vi "Change Password.vi"(8 "error in":errorcluster, 10 "New Password":string, 11 "User Name":string) -> (0 "error out":errorcluster)   [LabVIEW 2022 SP3]
uses:
  <vilib>/Utility/file.llb/Read Delimited Spreadsheet (string).vi
  <vilib>/Utility/file.llb/Write Delimited Spreadsheet (string).vi
panel:
  out "output array 2":string[](array[string])
  out "index of element":i32
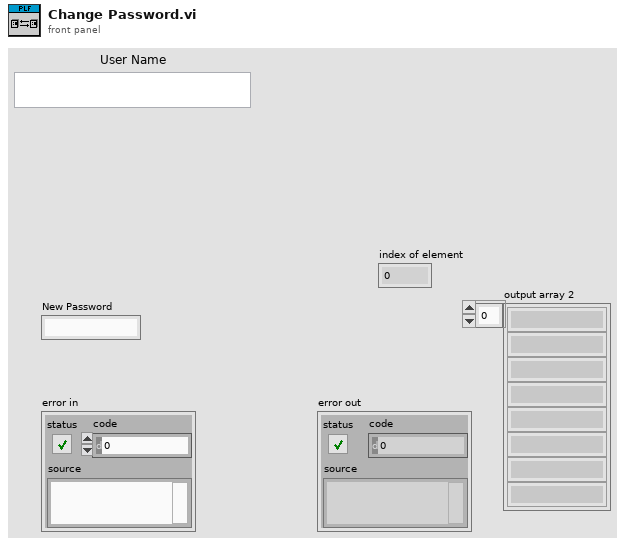
[diagram p1: front panel]
types:
  T1 = typedef "SeCrTs-file folder ctl.ctl" = cluster{"Datalog path":path, "Configuration path":path, "Signal list path":path, "Sub vi's":path, "Authentication":path, "Sequence":path, "Event Log":path, "CS Error log":path, "RT Error Log":path}
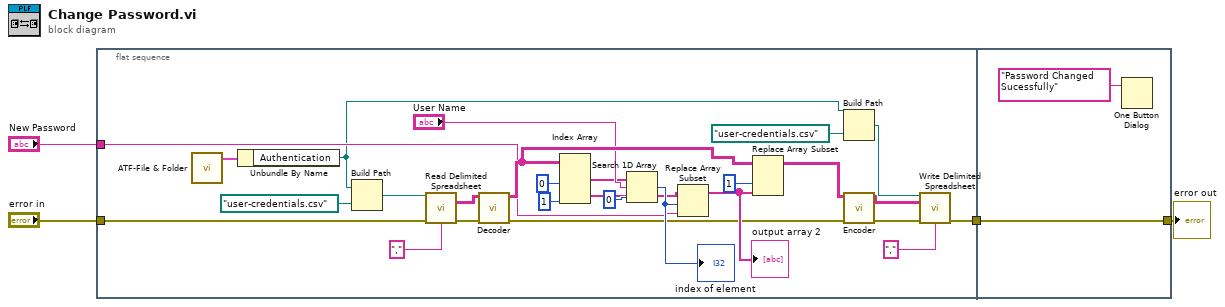
[diagram p0: block diagram]
diagram:
  n1 = flat-sequence {
    tunnel: "error in" -> [w18]
    tunnel: [w14] -> w4
    tunnel: "New Password" -> [w13]
    tunnel: [w33] -> w2
    tunnel: w4 -> [w33]
    frame #0 {
      n2 = call "ATF-File & Folder.vi"() -> ("File Output"=w6:T1)  [unwired: 10 in, 1 out]
      n3 = Unbundle By Name(w6) -> ("Authentication"=w5:path)
      n4 = Build Path(base path=w5, name or relative path=path "user-credentials.csv") -> (appended path=w26:path)
      n5 = call-poly <vilib>:"Read Delimited Spreadsheet.vi"("file path (dialog if empty)"=w26, "error in (no error)"=w18, "delimiter (\\t)"="," ("delimiter (\\t)")) -> ("all rows"=w31:string[][], "error out"=w17:errorcluster)  [unwired: 7 in, 4 out]
      n6 = call "Decoder.vi"("error in"=w17, "Encoded Data"=w31) -> ("error out"=w16:errorcluster, "Decoded Data"=w28:string[][])  [unwired: 8 in]
      n7 = Index Array(array=w28, index (col) #1=0 ("disabled index (col)"), index (col) #2=1 ("index (col)")) -> (element #1=w10:string[], element #2=w9:string[])  [unwired: 2 in]
      n8 = Search 1D Array(1D array=w10, element="User Name", start index (0)=0) -> (index of element=w27:i32)
      "index of element" <- w27
      n9 = Replace Array Subset(array=w9, new element=w13, index=w27) -> (w29:string[])
      "output array 2" <- w29
      n10 = Replace Array Subset(array=w28, new element=w29, index (col)=1 ("disabled index (col)")) -> (w30:string[][])  [unwired: 1 in]
      n11 = Build Path(base path=w5, name or relative path=path "user-credentials.csv") -> (appended path=w7:path)
      n12 = call "Encoder.vi"("error in"=w16, "Orginal Data"=w30) -> ("error Out"=w15:errorcluster, "Encoded Data"=w8:string[][])  [unwired: 8 in]
      n13 = call-poly <vilib>:"Write Delimited Spreadsheet.vi"("file path (dialog if empty)"=w7, "2D data"=w8, "error in (no error)"=w15, "delimiter (\\t)"="," ("delimiter (\\t)")) -> ("error out"=w14:errorcluster)  [unwired: 10 in, 1 out]
    }
    frame #1 {
      n14 = One Button Dialog(message="Password Changed Sucessfully") -> ()  [unwired: 1 in, 1 out]
    }
  }
  "error out" <- w2
